vi "Write Status.vi"(6 "Selector":T1, 8 "error in":errorcluster, 11 "MiniIO in":refnum<class "MiniIO.lvclass">) -> (0 "error out":errorcluster, 3 "MiniIO out":refnum<class "MiniIO.lvclass">)   [LabVIEW 2018, in "MiniIO.lvlib" / "MiniIO.lvclass"]
uses:
  MiniIO.lvclass
  PPLs/PLC/Parent/PLC.lvlibp/Custom Controls/Selector.ctl
  PPLs/PLC/Parent/PLC.lvlibp/PLC.lvclass
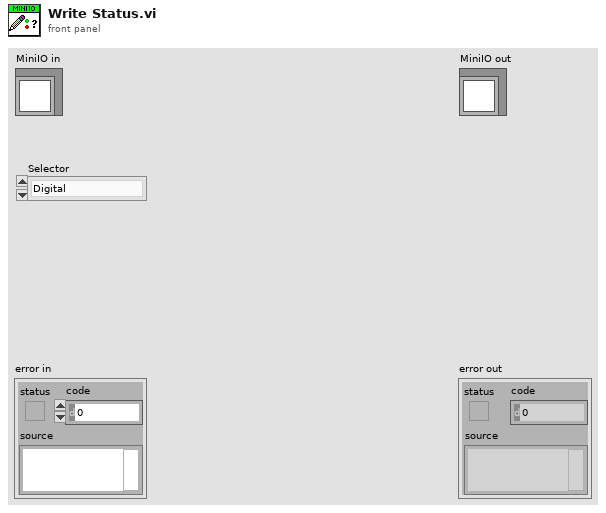
[diagram p1: front panel]
types:
  T1 = typedef "PLC.lvlibp/PLC.lvclass/Selector.ctl" = enum16{"Digital", "Analog"}
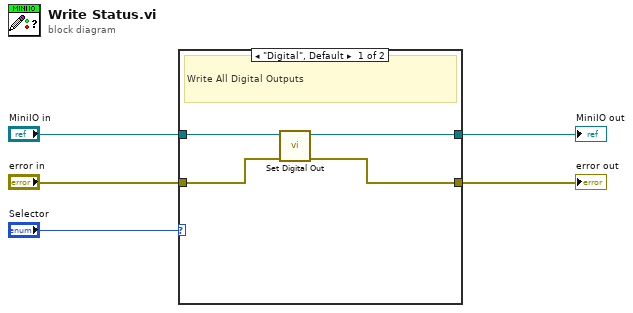
[diagram p0: block diagram]
diagram:
  n1 = case shown="\"Digital\", Default" "Selector" {
    tunnel: "error in" -> [w7 w10]
    tunnel: "MiniIO in" -> [w9 w11]
    tunnel: [w8 w11] -> w2
    tunnel: [w6 w10] -> w1
    frame "Digital", Default {
      # "Write All Digital Outputs"
      n2 = call "Set Digital Out.vi"("error in"=w7, "MiniIO in"=w9) -> ("error out"=w6:errorcluster, "MiniIO out"=w8:refnum<class "MiniIO.lvclass">)  [unwired: 8 in]
    }
    frame "Analog" {
      # "Mini IO does not have Analog IO"
    }
  }
  "error out" <- w1
  "MiniIO out" <- w2
